vi "Auto kicker.vi"(11 "Iteration":dbl) -> (2 "Stop":bool)   [LabVIEW 2017]
uses:
  Robot Global Data V.3.0.vi
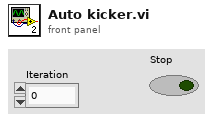
[diagram p1: front panel]
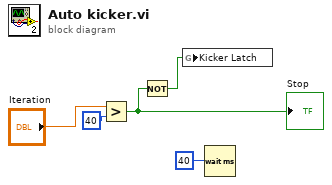
[diagram p0: block diagram]
diagram:
  n1 = Greater?(x="Iteration", y=40) -> (0:w2:bool)
  "Stop" <- w2
  n2 = Not(x=w2) -> (.not. x?=w3:bool)
  n3 = global write "Robot Global Data V.3.0.vi" "Kicker Latch"(w3) -> ()
  n4 = Wait (ms)(milliseconds to wait=u32 40) -> ()  [unwired: 1 out]
